vi "LVClass_Pupil Get Data.vi"(0 "Pupil in":refnum<class "Pupil.lvclass">, 11 "error in (no error)":errorcluster) -> (4 "Pupil out":refnum<class "Pupil.lvclass">, 6 "Data":i32[][](array[numeric]), 15 "error out":errorcluster)   [LabVIEW 2020, in "Pupil.lvclass"]
doc: "Get Pupil buffer.\n\n--------------------------------------------------------------------------------\n\n<B>PupilIn </B> : Pupil object.\n<B>PupilOut </B> : Pupil object.\n<B>data </B> : Pupil buffer.\n<B>ErrorIn </B> : Error\n<B>ErrorOut </B> : Error\n\n--------------------------------------------------------------------------------"
uses:
  Pupil.lvclass
  Pupil.lvclass/Pupil.ctl
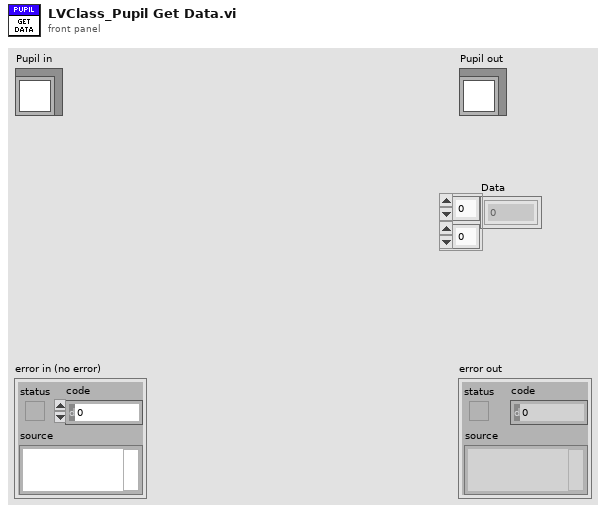
[diagram p1: front panel]
types:
  T1 = typedef "General dimensions definition.ctl" = cluster{"Size":T2, "Step":T3}
  T2 = typedef "Point2D.ctl" = cluster{"X":u32, "Y":u32}
  T3 = typedef "Point2Df.ctl" = cluster{"X":sgl, "Y":sgl}
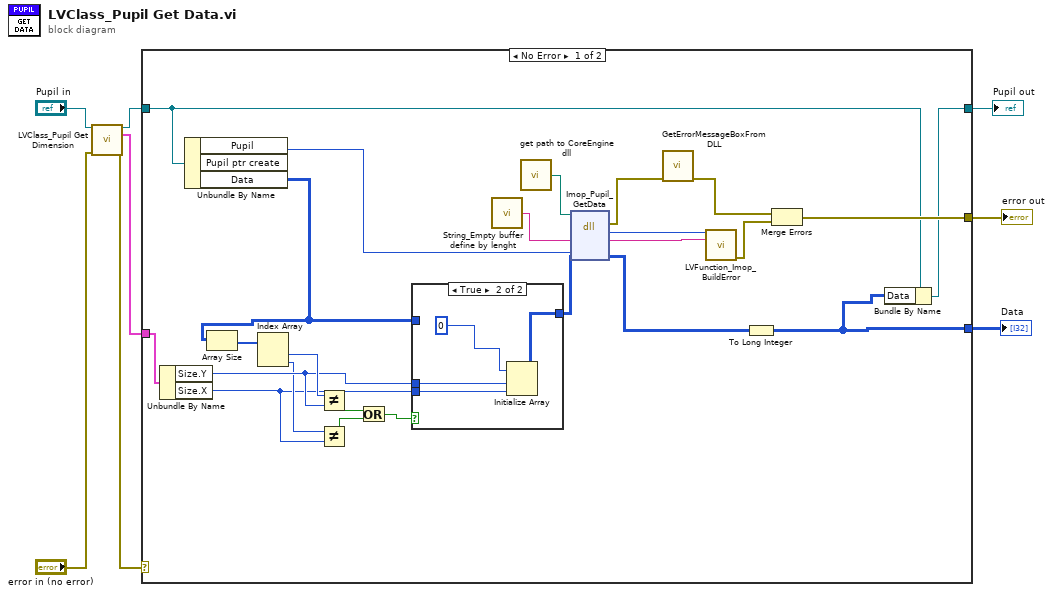
[diagram p0: block diagram]
diagram:
  n1 = call "LVClass_Pupil Get Dimension.vi"("Pupil in"="Pupil in", "error in (no error)"="error in (no error)") -> ("Pupil out"=w5:refnum<class "Pupil.lvclass">, "Dimension"=w4:T1, "error out"=w2:errorcluster)  [unwired: 11 in]
  n2 = case shown="No Error" w2 {
    selector: w2 -> [_ w39]
    tunnel: [w24 w39] -> w8
    tunnel: [w9 w38] -> w7
    tunnel: w5 -> [w10 w38]
    tunnel: w4 -> [w14 _]
    tunnel: [w11 _] -> w1
    frame No Error {
      n3 = Unbundle By Name(w14) -> ("Size.Y"=w20:u32, "Size.X"=w18:u32)
      n4 = Unbundle By Name(w10) -> ("Pupil"=w27:i32, "Data"=w13:i32[][])  [unwired: 1 out]
      n5 = Array Size(array=w13) -> (size(s)=w22:i32[])
      n6 = Index Array(array=w22) -> (element #1=w21:i32, element #2=w19:i32)  [unwired: 2 in]
      n7 = Not Equal?(x=w21, y=w20) -> (x != y?=w17:bool)
      n8 = Not Equal?(x=w19, y=w18) -> (x != y?=w16:bool)
      n9 = Or(x=w17, y=w16) -> (x .or. y?=w15:bool)
      n10 = case shown="True" w15 {
        tunnel: [w33 w35] -> w12
        tunnel: w20 -> [_ w37]
        tunnel: w18 -> [_ w36]
        tunnel: w13 -> [w33 _]
        frame False {
        }
        frame True {
          n11 = Initialize Array(u8 0, w37, w36) -> (w35:u8[][])
        }
      }
      n12 = call "String_Empty buffer define by lenght.vi"() -> ("Empty buffer"=w32:string)  [unwired: 1 in]
      n13 = call "get path to CoreEngine dll.vi"() -> ("path to c_interface_vc100.dll"=w29:path)  [unwired: 12 in, 3 out]
      n14 = dll-call lib="D:/2_trunk/Soft_haso/ImOpCoreEngine4_LV2011/DLLs/ImopEngine4_vc100.dll" fn="Imop_Pupil_GetData"(path in=w29, "message"=w32, "objet"=w27, "Data"=w12) -> (error out=w28:errorcluster, "return type"=w30:i32, "message"=w31:string, "Data"=w23:u8[][])  [unwired: 3 in, 1 out]
      n15 = call "GetErrorMessageBoxFromDLL.vi"("error IN"=w28) -> ("error OUT"=w26:errorcluster)  [unwired: 10 in]
      n16 = call "LVFunction_Imop_BuildError.vi"("code"=w30, "String to Prepend to source (\"\")"=w31) -> ("error out"=w25:errorcluster)  [unwired: 13 in]
      n17 = To Long Integer(number=w23) -> (32bit integer=w11:i32[][])
      n18 = Merge Errors(w26, w25) -> (w24:errorcluster)
      n19 = Bundle By Name(cluster=w10, "Data"=w11) -> (w9:refnum<class "Pupil.lvclass">)
    }
    frame Error {
    }
  }
  "error out" <- w8
  "Pupil out" <- w7
  "Data" <- w1
